vi "Acquire.vi"(8 "error in (no error)":errorcluster, 11 "Buffer in":refnum<class "Buffer.lvclass">) -> (0 "error out":errorcluster, 3 "Mapped Buffer":refnum<data-value>)   [LabVIEW 2020, in "Buffer Byte-Stream Access.lvclass"]
uses:
  Buffer Byte-Stream Access.lvclass
  Buffer/Buffer.lvclass
  Buffer/Buffer.lvclass/Buffer.ctl
  Image Info.ctl
  Buffer Byte-Stream Access.lvclass/Buffer Byte-Stream Access.ctl
  bin/gindustrialcam_32-1.dll
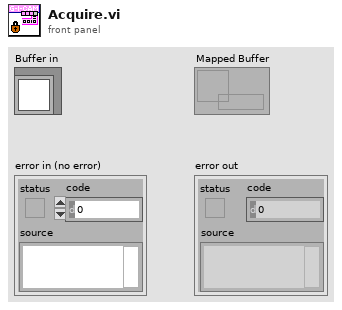
[diagram p1: front panel]
types:
  T1 = typedef "Buffer Byte-Stream Access.lvclass/Image Info.ctl" = cluster{"X Resolution":i32, "Y Resolution":i32, "Bytes to Copy":u64}
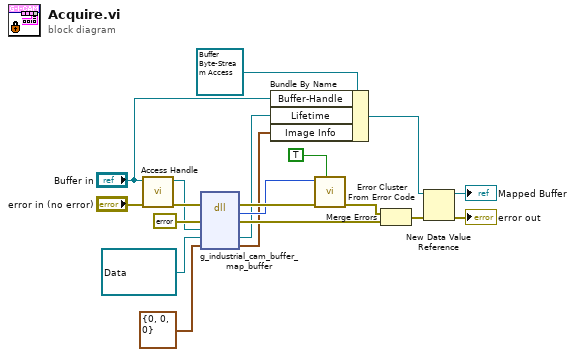
[diagram p0: block diagram]
diagram:
  n1 = call "Access Handle.vi"("error in (no error)"="error in (no error)", "Buffer"="Buffer in") -> ("error out"=w7:errorcluster, "Handle"=w6:refnum<data-value>)  [unwired: 8 in]
  n2 = dll-call lib="C:/serenial/lib/g-industrial-camera/LabVIEW/g_industrial_cam/bin/gindustrialcam_*-1.*" fn="g_industrial_cam_buffer_map_buffer"(error in=w7, "err"=errorcluster {"status"=FALSE, "code"=0, "source"=""} ("error constant"), "buffer_handle"=w6, "lifetime_edvr"=refnum<data-value> refnum ("Lifetime"), "info_ptr"=T1 {"X Resolution"=0, "Y Resolution"=0, "Bytes to Copy"=0} ("Image Info")) -> (error out=w13:errorcluster, "Mg_Error"=w12:i32, "err"=w10:errorcluster, "lifetime_edvr"=w4:refnum<data-value>, "info_ptr"=w2:T1)  [unwired: 3 in, 1 out]
  n3 = Bundle By Name(cluster=refnum<class "Buffer Byte-Stream Access.lvclass"> refnum ("Buffer-Mapped.lvclass"), "Buffer-Handle"="Buffer in", "Lifetime"=w4, "Image Info"=w2) -> (w17:refnum<class "Buffer Byte-Stream Access.lvclass">)
  n4 = call <vilib>:"Error Cluster From Error Code.vi"("show call chain? (False)"=TRUE, "error in (no error)"=w13, "error code (0)"=w12) -> ("error out"=w11:errorcluster)  [unwired: 6 in]
  n5 = Merge Errors(w11, w10) -> (w1:errorcluster)
  n6 = New Data Value Reference(data value=w17, error in=w1) -> (data value reference=→"Mapped Buffer":refnum<data-value>, error out=→"error out":errorcluster)
